vi "Display and Log Process.vi"(8 "Parameters":variant, 11 "Process":refnum<class "Process.lvclass">) -> ()   [LabVIEW 2024, in "VS Plugin Inline Async API.lvlib"]
uses:
  VS Plugin Inline Async API.lvlib
  <vilib>/NI VeriStand/Custom Device Tools/Custom Device Utility Library/Custom Device Utility Library.lvlib
  <vilib>/Utility/SystemLogging/NI_SystemLogging.lvlib
  Process/Process.lvclass
  VS Plugin Inline Async API/Types/Error Handling Settings.ctl
  VS Plugin Inline Async API/VS Plugin Inline Async API.lvclass
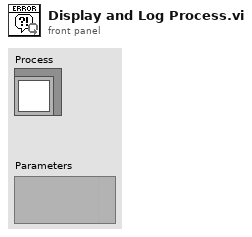
[diagram p1: front panel]
types:
  T1 = typedef "VS Plugin Inline Async API.lvlib/VS Plugin Inline Async API.lvclass/Error Handling Settings.ctl" = cluster{"Write to SystemLog (F)":bool}
  T2 = cluster{"read mode":enum16{"polling", "blocking"}, "write mode":enum16{"polling", "blocking"}}
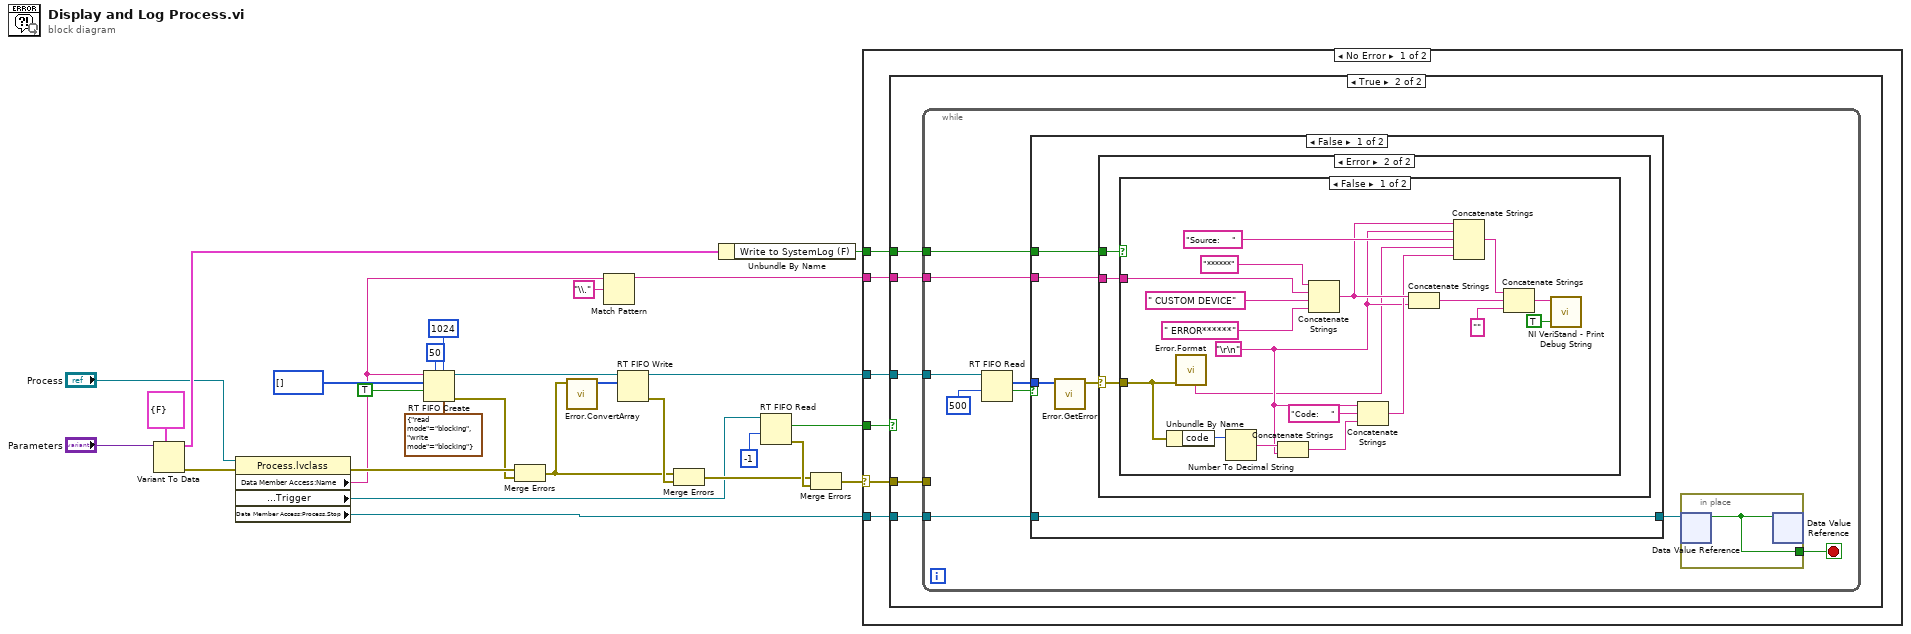
[diagram p0: block diagram]
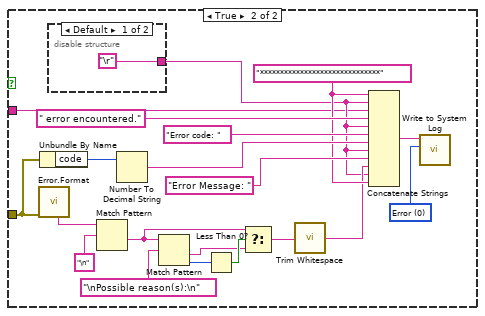
[diagram p4: hidden frame]
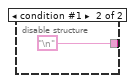
[diagram p5: hidden frame]
diagram:
  n1 = Variant To Data(type=T1 {"Write to SystemLog (F)"=FALSE}, Variant="Parameters") -> (data=w7:T1, error out=w21:errorcluster)  [unwired: 1 in]
  n2 = property class="Process.lvclass"(reference="Process", error in=w21) -> (error out=w28:errorcluster, "Data Member Access:Name"=w5:string, "Data Member Access:Process.Trigger"=w11:refnum<k33>, "Data Member Access:Process.Stop"=w19:refnum<data-value>)  [unwired: 1 out]
  n3 = RT FIFO Create(0:w5, 1:u8[] [], 2:TRUE ("create if not found? (T)"), 4:u32 50 ("size (10)"), 6:u32 1024 ("elements in array (1)"), 7:T2 {"read mode"=enum."blocking", "write mode"=enum."blocking"} ("r/w modes (polling,polling)")) -> (8:w20:refnum<k33>, 11:w26:errorcluster)  [unwired: 2 in, 1 out]
  n4 = Merge Errors(w28, w26) -> (w25:errorcluster)
  n5 = call "Error.ConvertArray.vi"("error in"=w25) -> ("Msg"=w16:u8[])  [unwired: 10 in]
  n6 = Match Pattern(string=w5, regular expression="\\.") -> (before substring=w4:string)  [unwired: 1 in, 3 out]
  n7 = RT FIFO Write(0:w20, 1:w16) -> (8:w9:refnum<k33>, 11:w27:errorcluster)  [unwired: 3 in, 2 out]
  n8 = Merge Errors(w25, w27) -> (w23:errorcluster)
  n9 = Unbundle By Name(w7) -> ("Write to SystemLog (F)"=w6:bool)
  n10 = RT FIFO Read(0:w11, 2:-1 ("timeout in ms (-1)")) -> (9:w10:bool, 11:w24:errorcluster)  [unwired: 2 in, 3 out]
  n11 = Merge Errors(w23, w24) -> (w22:errorcluster)
  n12 = case shown="No Error" w22 {
    selector: w22 -> [w34 _]
    tunnel: w10 -> [w33 _]
    tunnel: w4 -> [w32 _]
    tunnel: w9 -> [w31 _]
    tunnel: w19 -> [w30 _]
    tunnel: w6 -> [w29 _]
    frame No Error {
      n13 = case shown="True" w33 {
        tunnel: w31 -> [_ w38]
        tunnel: w32 -> [_ w37]
        tunnel: w34 -> [_ w39]
        tunnel: w30 -> [_ w36]
        tunnel: w29 -> [_ w35]
        frame False {
        }
        frame True {
          n14 = while {
            tunnel: w38 -> [w48]
            tunnel: w37 -> [w47]
            tunnel: w39 -> [_]
            tunnel: w36 -> [w41]
            tunnel: w35 -> [w40]
            stop <- w43 stop-if-true
            n15 = RT FIFO Read(0:w48, 2:500 ("timeout in ms (-1)")) -> (9:w46:u8[], 10:w44:bool)  [unwired: 2 in, 3 out]
            n16 = case shown="False" w44 {
              tunnel: w46 -> [w52 _]
              tunnel: w47 -> [w51 _]
              tunnel: [w53 w99] -> w42
              tunnel: w41 -> [w53 w99]
              tunnel: w40 -> [w50 _]
              frame False {
                n17 = call "Error.GetError.vi"("Msg"=w52) -> ("error out"=w54:errorcluster)  [unwired: 10 in]
                n18 = case shown="Error" w54 {
                  selector: w54 -> [_ w57]
                  tunnel: w51 -> [_ w56]
                  tunnel: w50 -> [_ w55]
                  frame No Error {
                  }
                  frame Error {
                    n19 = case shown="False" w55 {
                      tunnel: w56 -> [w63 w79]
                      tunnel: w57 -> [w76 w96]
                      frame False {
                        w62 = "\r\n"
                        n20 = Unbundle By Name(w76) -> ("code"=w65:i32)
                        n21 = call "Error.Format.vi"("error in"=w76) -> ("message"=w58:string)  [unwired: 6 in, 4 out]
                        n22 = Number To Decimal String(number=w65) -> (decimal integer string=w73:string)  [unwired: 1 in]
                        n23 = Concatenate Strings(w73, w62) -> (w64:string)
                        n24 = Concatenate Strings("******" ("String"), w63, " CUSTOM DEVICE" ("String"), " ERROR******" ("String")) -> (w70:string)
                        n25 = Concatenate Strings(w62, "Code:    " ("String"), w64) -> (w69:string)
                        n26 = Concatenate Strings(w70, w62) -> (w67:string)
                        n27 = Concatenate Strings(w70, w62, "Source:    " ("String"), w58, w69) -> (w68:string)
                        n28 = Concatenate Strings(w68, w67, "" ("Message")) -> (w61:string)
                        n29 = call <vilib>:"NI VeriStand - Print Debug String.vi"("Add to log file? (F)"=TRUE ("Add to log file? (T)"), "Message"=w61) -> ()  [unwired: 9 in, 1 out]
                      }
                      frame True {
                        w90 = "******************************" ("string")
                        w95 = 0 items=["Error", "Warning", "Informational"] ("severity")
                        n30 = call "Error.Format.vi"("error in"=w96) -> ("message"=w77:string)  [unwired: 6 in, 4 out]
                        n31 = Unbundle By Name(w96) -> ("code"=w78:i32)
                        n32 = disable-structure shown="Default" {
                          disable-tunnel: ["\r" "\n"] -> w81
                          frame condition #0 (active) {
                          }
                          frame condition #1 {
                          }
                        }
                        n33 = Match Pattern(string=w77, regular expression="\n" ("string")) -> (after substring=w85:string)  [unwired: 1 in, 3 out]
                        n34 = Number To Decimal String(number=w78) -> (decimal integer string=w92:string)  [unwired: 1 in]
                        n35 = Match Pattern(string=w85, regular expression="\nPossible reason(s):\n" ("string")) -> (after substring=w84:string, offset past match=w87:i32)  [unwired: 1 in, 2 out]
                        n36 = Less Than 0?(x=w87) -> (x < 0?=w86:bool)
                        n37 = Select(t=w85, s=w86, f=w84) -> (s? t:f=w83:string)
                        n38 = call <vilib>:"Trim Whitespace.vi"("string"=w83) -> ("trimmed string"=w82:string)  [unwired: 1 in]
                        n39 = Concatenate Strings(w90, w81, w79, " error encountered." ("String"), w81, "Error code: " ("string"), w92, w81, "Error Message: " ("string"), w82, w81, w90) -> (w80:string)
                        n40 = call <vilib>:"Write to System Log.vi"("severity"=w95, "message"=w80) -> ()  [unwired: 9 in, 1 out]
                      }
                    }
                  }
                }
              }
              frame True {
              }
            }
            n41 = in-place {
              in-place-border: [w49] -> w43
              n42 = in-place-dvr #1(w42) -> (w49:bool)  [unwired: 1 out]
              n43 = in-place-dvr #1(w49) -> ()  [unwired: 2 out]
            }
          }
        }
      }
    }
    frame Error {
    }
  }
